vi "Simulate Temperature.vi"(10 "Delta T":dbl=0.01, 11 "Starting Temp":dbl=80.0) -> (3 "Temp (F)":dbl)   [LabVIEW 2017, in "Library.lvlib"]
doc: "Generates a random tempture. The starting temperature is the starting tempurature. The Delta T manages how much the temperature can change (by %) by in 1 iteration."
uses:
  Library.lvlib
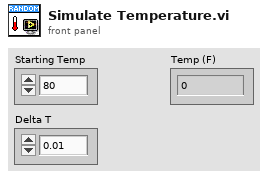
[diagram p1: front panel]
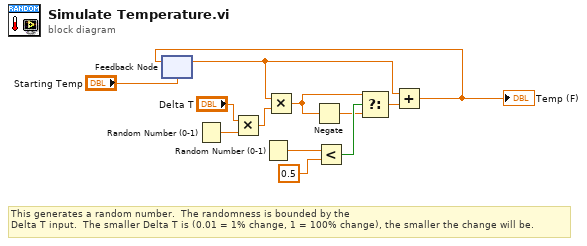
[diagram p0: block diagram]
diagram:
  # "This generates a random number.  The randomness is bounded by the\nDelta T input.  The smaller Delta T is (0.01 = 1% change, 1 = 100% change), the smaller the change will be."
  n1 = feedback #1("Starting Temp") -> (w2:dbl)
  n2 = Random Number (0-1)() -> (number: 0 to 1=w12:dbl)
  n3 = Multiply(x="Delta T", y=w12) -> (x*y=w10:dbl)
  n4 = Random Number (0-1)() -> (number: 0 to 1=w9:dbl)
  n5 = Multiply(x=w2, y=w10) -> (x*y=w5:dbl)
  n6 = Negate(x=w5) -> (-x=w6:dbl)
  n7 = Less?(x=w9, y=0.5) -> (x < y?=w7:bool)
  n8 = Select(t=w5, s=w7, f=w6) -> (s? t:f=w4:dbl)
  n9 = Add(x=w2, y=w4) -> (x+y=w1:dbl)
  "Temp (F)" <- w1
  n10 = feedback-in #1(w1) -> ()
